vi "Fetch PRACH Sequence Correlation Results.vi"(8 "error in (no error)":errorcluster, 10 "Instance (1)":T1=1, 11 "VISA resource name":refnum<visa-resource-name>) -> (0 "error out":errorcluster, 1 "Result":dbl format="%^.3e", 2 "Reliability":i32, 3 "VISA resource name out":refnum<visa-resource-name>)   [LabVIEW 2020, in "Rohde&Schwarz CMWXP NR FR1 Measurement.lvlib"]
doc: "Returns the sequence correlation for single-preamble measurements. It indicates the correlation between the ideal preamble sequence determined from the parameter settings and the measured preamble sequence. A value of 1 corresponds to perfect correlation. A value much smaller than 1 indicates that the preamble sequence was not found.\n\nAttribute:\nRSCMWXPNRFR1M_ATTR_FETCH_PRACH_SEQUENCE_CORRELATION_RESULTS\n\nRemote-control command:\nFETCh:NRSub:MEAS<i>:PRACh:MODulation:SCORrelation?"
uses:
  <instrlib>/Rohde&Schwarz CMWXP NR FR1 Measurement/Rohde&Schwarz CMWXP NR FR1 Measurement.lvlib
  <instrlib>/Rohde&Schwarz CMWXP NR FR1 Measurement/Private/_Instance.ctl
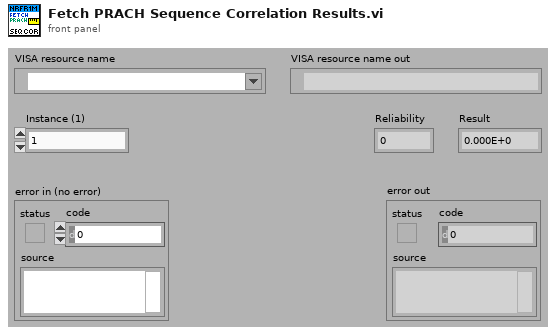
[diagram p1: front panel]
types:
  T1 = typedef "Rohde&Schwarz CMWXP NR FR1 Measurement.lvlib/_Instance.ctl" = i32
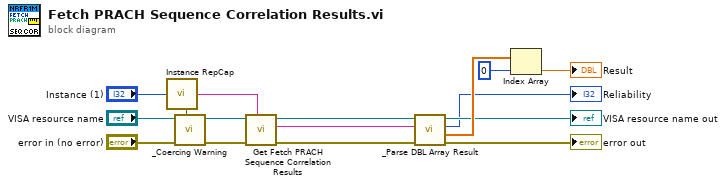
[diagram p0: block diagram]
diagram:
  n1 = call <instrlib>:"Instance RepCap.vi"("Instance In"="Instance (1)") -> ("In Range?"=w11:bool, "RepCap Identifier Out"=w10:string)  [unwired: 1 in]
  n2 = call <instrlib>:"_Coercing Warning.vi"("In Range?"=w11, "error in (no error)"="error in (no error)", "VISA resource name"="VISA resource name") -> ("error out"=w14:errorcluster, "VISA resource name out"=w13:refnum<visa-resource-name>)  [unwired: 7 in]
  n3 = call "Get Fetch PRACH Sequence Correlation Results"("Repeated Capabilities"=w10, "error in (no error)"=w14, "instrument handle"=w13) -> ("error out"=w2:errorcluster, "Fetch PRACH Sequence Correlation Results"=w5:string, "instrument handle out"=w7:refnum<visa-resource-name>)  [unwired: 6 in]
  n4 = call <instrlib>:"_Parse DBL Array Result.vi"("error in (no error)"=w2, "Input String"=w5, "VISA resource name"=w7) -> ("error out"=→"error out":errorcluster, "Results"=w8:dbl[], "Reliability"=→"Reliability":i32, "VISA resource name out"=→"VISA resource name out":refnum<visa-resource-name>)  [unwired: 5 in]
  n5 = Index Array(array=w8, index=0) -> (element=→"Result":dbl)
